vi "IsSlaveActive.vi"(10 "Active slaves":T2, 11 "Enum":T1) -> (3 "camera":bool)   [LabVIEW 2018, in "MasterProgramSupportFunctions.lvlib"]
uses:
  MasterProgramSupportFunctions.lvlib
  ActiveSlaves.ctl
  VI_tags.ctl
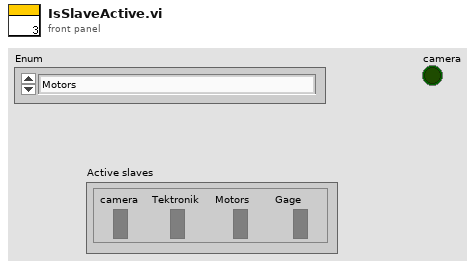
[diagram p1: front panel]
types:
  T1 = typedef "MasterProgramSupportFunctions.lvlib/VI_tags.ctl" = enum16{"Motors", "Gage", "Tektro3107", "XimeaMainCamera", "ContinuousMainScan"}
  T2 = typedef "MasterProgramSupportFunctions.lvlib/ActiveSlaves.ctl" = cluster{"camera":bool, "Tektronik":bool, "Motors":bool, "Gage":bool}
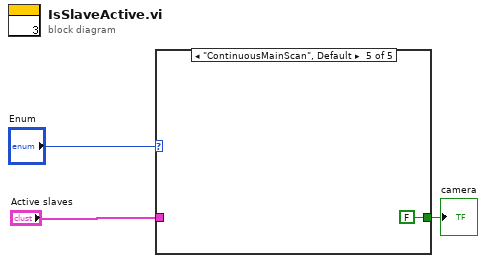
[diagram p0: block diagram]
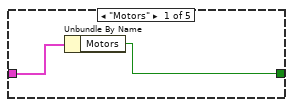
[diagram p2: hidden frame]
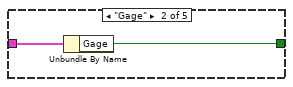
[diagram p3: hidden frame]
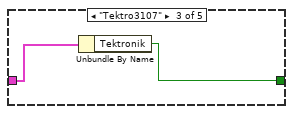
[diagram p4: hidden frame]
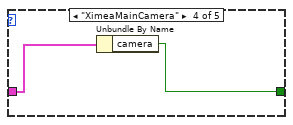
[diagram p5: hidden frame]
diagram:
  n1 = case shown="\"ContinuousMainScan\", Default" "Enum" {
    tunnel: "Active slaves" -> [w5 w7 w9 w11 _]
    tunnel: [w4 w6 w8 w10 FALSE ("Gage")] -> w1
    frame "Motors" {
      n2 = Unbundle By Name(w5) -> ("Motors"=w4:bool)
    }
    frame "Gage" {
      n3 = Unbundle By Name(w7) -> ("Gage"=w6:bool)
    }
    frame "Tektro3107" {
      n4 = Unbundle By Name(w9) -> ("Tektronik"=w8:bool)
    }
    frame "XimeaMainCamera" {
      n5 = Unbundle By Name(w11) -> ("camera"=w10:bool)
    }
    frame "ContinuousMainScan", Default {
    }
  }
  "camera" <- w1
